vi "Layer3_ReceiveResponse.vi"(8 "Error In":errorcluster, 11 "Serial Port to Use":refnum<visa-resource-name>="COM8") -> (1 "Response Message":string, 2 "Response CMD":u16, 3 "Message Received":bool, 4 "Error Out":errorcluster, 5 "Serial Port to Use (out)":refnum<visa-resource-name>)   [LabVIEW 2012]
uses:
  Arduino_Serial_GlobalConstants.vi
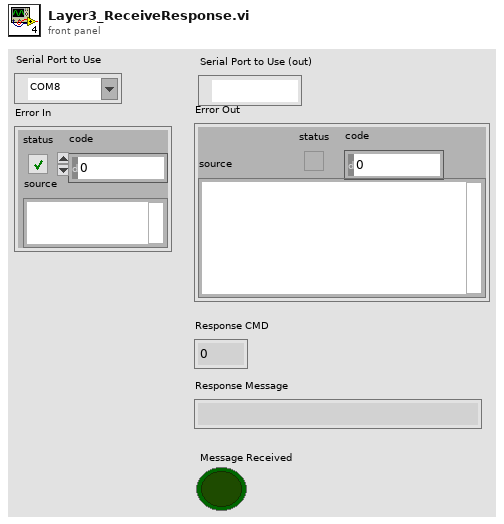
[diagram p1: front panel]
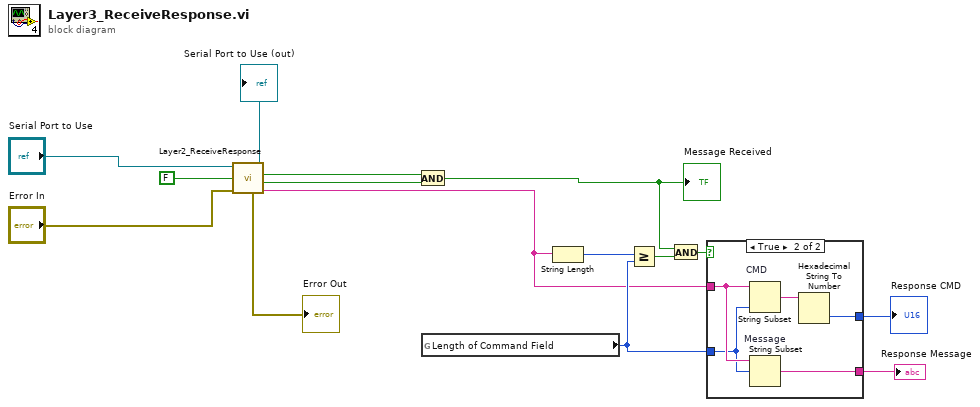
[diagram p0: block diagram]
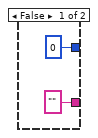
[diagram p2: hidden frame]
diagram:
  n1 = call "Layer2_ReceiveResponse.vi"("Error In"="Error In", "Expecting Response"=FALSE, "Serial Port to Use"="Serial Port to Use") -> ("Layer2 Payload"=w4:string, "No Errors"=w1:bool, "Response Received"=w2:bool, "Error Out"=→"Error Out":errorcluster, "Serial Port to Use (out)"=→"Serial Port to Use (out)":refnum<visa-resource-name>)  [unwired: 3 in, 1 out]
  n2 = And(x=w2, y=w1) -> (x .and. y?=w3:bool)
  "Message Received" <- w3
  n3 = global read "Arduino_Serial_GlobalConstants.vi" "Length of Command Field"() -> (w12:i32)
  n4 = String Length(string=w4) -> (length=w13:i32)
  n5 = Greater Or Equal?(x=w13, y=w12) -> (x >= y?=w10:bool)
  n6 = And(x=w3, y=w10) -> (x .and. y?=w11:bool)
  n7 = case shown="True" w11 {
    tunnel: w4 -> [_ w21]
    tunnel: w12 -> [_ w20]
    tunnel: [u32 0 w19] -> w15
    tunnel: ["" ("Layer2 Payload") w18] -> w14
    frame False {
    }
    frame True {
      n8 = String Subset "CMD"(string=w21, length (rest)=w20) -> (substring=w22:string)  [unwired: 1 in]
      n9 = String Subset "Message"(string=w21, offset (0)=w20) -> (substring=w18:string)  [unwired: 1 in]
      n10 = Hexadecimal String To Number(string=w22) -> (number=w19:u32)  [unwired: 2 in, 1 out]
    }
  }
  "Response Message" <- w14
  "Response CMD" <- w15
